vi "ListenNewClientsConnections.vi"(8 "error in (no error)":errorcluster, 10 "Port":i32=6341, 11 "NetworkClient in":refnum<class "NetworkServer.lvclass">) -> (0 "error out":errorcluster, 3 "NetworkClient out":refnum<class "NetworkServer.lvclass">)   [LabVIEW 2011, in "Hardware.lvlib" / "HWControllers.lvlib" / "NetworkServer.lvclass"]
uses:
  NetworkServer.lvclass
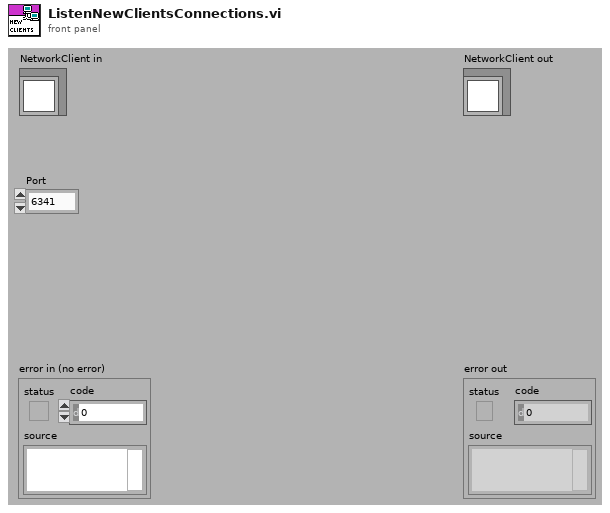
[diagram p1: front panel]
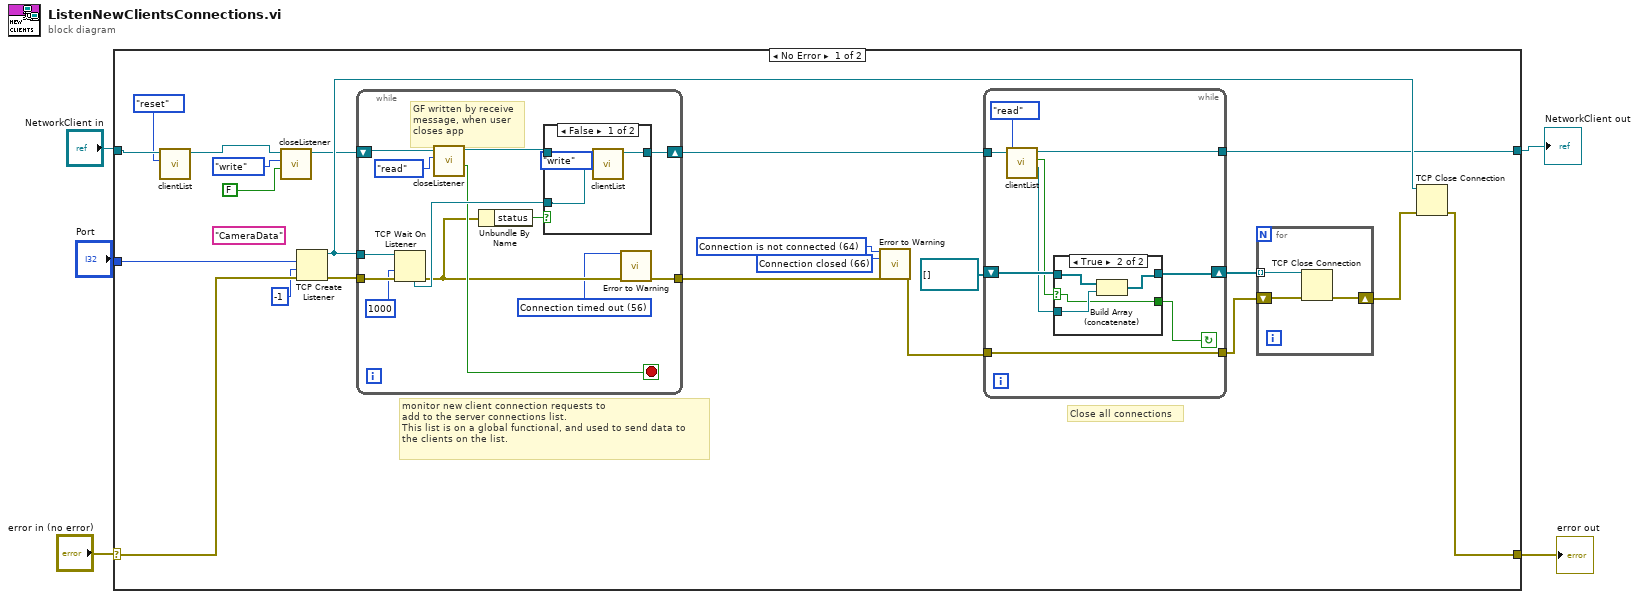
[diagram p0: block diagram]
diagram:
  n1 = case shown="No Error" "error in (no error)" {
    selector: "error in (no error)" -> [w16 w65]
    tunnel: [w19 w65] -> w4
    tunnel: [w13 w64] -> w3
    tunnel: "NetworkClient in" -> [w8 w64]
    tunnel: "Port" -> [w15 _]
    frame No Error {
      (unwired) "CameraData" ("service name")
      w25 = 66 items=["No Error", "Argument Error", "Memory Full", "Out of Zone", "End of File", "File Already Open", "Generic File IO Error", "File Not Found", "File Permission Error", "Disk Full", "Duplicate Path", "Too Many Files Open", "Not Enabled", "Resource File Not Found", "Cannot Add Resource", "Resource Not Found", "Image Not Found", "Image Memory Error", "Pen Does Not Exist", "Config Bad Type", "Config Token Not Found", "Config Parse Error", "Config Memory Error", "Bad External Code Format", "Bad External Code Offset", "External Code Not Present", "Null Window", "Destroy Window Mixup", "Null Menu", "Print Aborted", "Bad Print Record", "Print Driver Error", "Windows Error During Print", "Memory Error During Print", "Print Dialog Error", "Generic Print Error", "Invalid Device Refnum", "Device Not Found", "Device Parameter Error", "Device Unit Error", "Can't Open Device", "Device Call Aborted", "Generic Error", "Cancelled By User", "Object ID Too Low", "Object ID Too High", "Object Not In Heap", "Unknown Heap", "Bad DefProc ID", "DefProc Not In Table", "Message Out Of Range", "Null Method", "Unknown Message", "Manager Call Not Supported", "Bad address", "Connection In progress", "Connection timed out", "Connection is already in progress", "Network attribute not supported", "Network error", "Address in use", "System out of memory", "Connection aborted", "Connection refused", "Connection is not connected", "Connection is already connected", "Connection closed", "Initialize error (interapplication manager)", "Bad occurrence", "Wait on unbound occurrence handler", "Occurrence queue overflow", "Bad path", "Semaphore not signaled", "Unrecognized type (interapplication manager)"] ("2nd Error to Convert")
      w26 = 64 items=["No Error", "Argument Error", "Memory Full", "Out of Zone", "End of File", "File Already Open", "Generic File IO Error", "File Not Found", "File Permission Error", "Disk Full", "Duplicate Path", "Too Many Files Open", "Not Enabled", "Resource File Not Found", "Cannot Add Resource", "Resource Not Found", "Image Not Found", "Image Memory Error", "Pen Does Not Exist", "Config Bad Type", "Config Token Not Found", "Config Parse Error", "Config Memory Error", "Bad External Code Format", "Bad External Code Offset", "External Code Not Present", "Null Window", "Destroy Window Mixup", "Null Menu", "Print Aborted", "Bad Print Record", "Print Driver Error", "Windows Error During Print", "Memory Error During Print", "Print Dialog Error", "Generic Print Error", "Invalid Device Refnum", "Device Not Found", "Device Parameter Error", "Device Unit Error", "Can't Open Device", "Device Call Aborted", "Generic Error", "Cancelled By User", "Object ID Too Low", "Object ID Too High", "Object Not In Heap", "Unknown Heap", "Bad DefProc ID", "DefProc Not In Table", "Message Out Of Range", "Null Method", "Unknown Message", "Manager Call Not Supported", "Bad address", "Connection In progress", "Connection timed out", "Connection is already in progress", "Network attribute not supported", "Network error", "Address in use", "System out of memory", "Connection aborted", "Connection refused", "Connection is not connected", "Connection is already connected", "Connection closed", "Initialize error (interapplication manager)", "Bad occurrence", "Wait on unbound occurrence handler", "Occurrence queue overflow", "Bad path", "Semaphore not signaled", "Unrecognized type (interapplication manager)"] ("1st Error to Convert")
      # "Close all connections"
      # "monitor new client connection requests to \nadd to the server connections list.\nThis list is on a global functional, and used to send data to\nthe clients on the list."
      n2 = call "clientList.vi"("Enum"=enum16{"read", "write", "reset"}."reset", "NetworkServer in"=w8) -> ("NetworkServer out"=w9:refnum<class "NetworkServer.lvclass">)  [unwired: 6 in, 3 out]
      n3 = call "closeListener.vi"("close"=FALSE, "actions"=enum16{"read", "write"}."write", "NetworkServer in"=w9) -> ("NetworkServer out"=w11:refnum<class "NetworkServer.lvclass">)  [unwired: 6 in, 2 out]
      n4 = TCP Create Listener(8:w16, 9:-1, 10:w15) -> (0:w18:errorcluster, 3:w17:refnum<k5>)  [unwired: 2 in, 1 out]
      n5 = while "Listen loop.  Append new connections to a synchronized queue." {
        tunnel: w17 -> [w57]
        tunnel: w18 -> [w58]
        tunnel: [w48] -> w27
        shift-right: [w54] -> w14
        shift-left: w11 -> [w53]
        stop <- w51 stop-if-true
        w46 = 56 items=["No Error", "Argument Error", "Memory Full", "Out of Zone", "End of File", "File Already Open", "Generic File IO Error", "File Not Found", "File Permission Error", "Disk Full", "Duplicate Path", "Too Many Files Open", "Not Enabled", "Resource File Not Found", "Cannot Add Resource", "Resource Not Found", "Image Not Found", "Image Memory Error", "Pen Does Not Exist", "Config Bad Type", "Config Token Not Found", "Config Parse Error", "Config Memory Error", "Bad External Code Format", "Bad External Code Offset", "External Code Not Present", "Null Window", "Destroy Window Mixup", "Null Menu", "Print Aborted", "Bad Print Record", "Print Driver Error", "Windows Error During Print", "Memory Error During Print", "Print Dialog Error", "Generic Print Error", "Invalid Device Refnum", "Device Not Found", "Device Parameter Error", "Device Unit Error", "Can't Open Device", "Device Call Aborted", "Generic Error", "Cancelled By User", "Object ID Too Low", "Object ID Too High", "Object Not In Heap", "Unknown Heap", "Bad DefProc ID", "DefProc Not In Table", "Message Out Of Range", "Null Method", "Unknown Message", "Manager Call Not Supported", "Bad address", "Connection In progress", "Connection timed out", "Connection is already in progress", "Network attribute not supported", "Network error", "Address in use", "System out of memory", "Connection aborted", "Connection refused", "Connection is not connected", "Connection is already connected", "Connection closed", "Initialize error (interapplication manager)", "Bad occurrence", "Wait on unbound occurrence handler", "Occurrence queue overflow", "Bad path", "Semaphore not signaled", "Unrecognized type (interapplication manager)"] ("1st Error to Convert")
        # "GF written by receive\nmessage, when user\ncloses app"
        n6 = TCP Wait On Listener(8:w58, 9:1000, 11:w57) -> (0:w47:errorcluster, 4:w56:refnum<k5>)  [unwired: 4 out]
        n7 = call "closeListener.vi"("actions"=enum16{"read", "write"}."read", "NetworkServer in"=w53) -> ("close"=w51:bool, "NetworkServer out"=w52:refnum<class "NetworkServer.lvclass">)  [unwired: 7 in, 1 out]
        n8 = Unbundle By Name(w47) -> ("status"=w55:bool)
        n9 = case shown="False" w55 {
          tunnel: w56 -> [w60 _]
          tunnel: w52 -> [w62 w63]
          tunnel: [w61 w63] -> w54
          frame False {
            n10 = call "clientList.vi"("new client"=w60, "Enum"=enum16{"read", "write", "reset"}."write", "NetworkServer in"=w62) -> ("NetworkServer out"=w61:refnum<class "NetworkServer.lvclass">)  [unwired: 5 in, 3 out]
          }
          frame True {
          }
        }
        n11 = call <vilib>:"Error to Warning.vi"("1st Error to Convert"=w46, "error in"=w47) -> ("warning out"=w48:errorcluster)  [unwired: 3 in, 10 out]
      }
      n12 = call <vilib>:"Error to Warning.vi"("1st Error to Convert"=w26, "2nd Error to Convert"=w25, "error in"=w27) -> ("warning out"=w21:errorcluster)  [unwired: 2 in, 10 out]
      n13 = while {
        shift-right: [w37] -> w23
        shift-left: refnum<k5>[] [] ("empty") -> [w38]
        tunnel: w21 -> [w36]
        tunnel: [w36] -> w22
        tunnel: w14 -> [w35]
        tunnel: [w34] -> w13
        stop <- w39 continue-if-true
        n14 = call "clientList.vi"("Enum"=enum16{"read", "write", "reset"}."read", "NetworkServer in"=w35) -> ("client"=w32:refnum<k5>, "valid?"=w33:bool, "NetworkServer out"=w34:refnum<class "NetworkServer.lvclass">)  [unwired: 6 in, 1 out]
        n15 = case shown="True" w33 {
          selector: w33 -> [w40 w43]
          tunnel: w32 -> [_ w45]
          tunnel: w38 -> [w41 w44]
          tunnel: [w40 w43] -> w39
          tunnel: [w41 w42] -> w37
          frame False {
          }
          frame True {
            n16 = Build Array (concatenate)(w44, w45) -> (w42:refnum<k5>[])
          }
        }
      }
      n17 = for {
        tunnel: w23 -> [w30] mode=indexing
        shift-right: [w29] -> w20
        shift-left: w22 -> [w28]
        n18 = TCP Close Connection(connection ID=w30, error in (no error)=w28) -> (error out=w29:errorcluster)  [unwired: 1 in, 1 out]
      }
      n19 = TCP Close Connection(connection ID=w17, error in (no error)=w20) -> (error out=w19:errorcluster)  [unwired: 2 out]
    }
    frame Error {
    }
  }
  "error out" <- w4
  "NetworkClient out" <- w3
